vi "Set Module Configuration.vi"(8 "error in (no error)":errorcluster, 10 "Configuration":T2, 11 "Data Cluster":T1) -> (0 "error out":errorcluster, 3 "Data Cluster dup":T1)   [LabVIEW 2014, in "Configurable.lvlib"]
uses:
  Configurable.lvlib
  ModuleConfiguration--Cluster.ctl
  Module Data--cluster.ctl
  <vilib>/LabVIEW Open Source/Configuration Manager/Manager/ConfigManager.lvclass
  <vilib>/LabVIEW Open Source Project/Unicity/UniqueName/UniqueNameClass/UniqueName.lvclass
  <vilib>/LabVIEW Open Source Project/Unicity/UniqueName/UniqueNameClass/UniqueName.lvclass/UniqueName.ctl
  <vilib>/LabVIEW Open Source/Configuration Manager/Manager/ConfigManager.lvclass/ConfigManager.ctl
  <vilib>/LabVIEW Open Source/Configuration Manager/Manager/Write.vi
  <vilib>/LabVIEW Open Source/Configuration Manager/Manager/Read Serializer.vi
  <vilib>/LabVIEW Open Source/Configuration Manager/Manager/Read Encoding.vi
  <vilib>/LabVIEW Open Source/Configuration Manager/Manager/Read Encryption.vi
  <vilib>/LabVIEW Open Source/Configuration Manager/Manager/Decompose KVPs.vi
  <vilib>/Utility/VariantDataType/GetTypeInfo.vi
  <vilib>/LabVIEW Open Source/Configuration Manager/Cache/ConfigManager.Cache.lvclass
  <vilib>/LabVIEW Open Source/Configuration Manager/Serializer/Serializer.lvclass
  <vilib>/LabVIEW Open Source/Configuration Manager/Encoding/Encoding.lvclass
  <vilib>/LabVIEW Open Source/Configuration Manager/Encryption/Encryption.lvclass
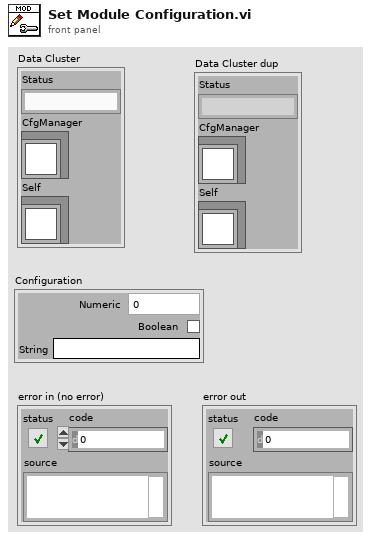
[diagram p1: front panel]
types:
  T1 = typedef "Configurable.lvlib/Module Data--cluster.ctl" = cluster{"Status":string, "CfgManager":refnum<class "ConfigManager.lvclass">, "Self":refnum<class "UniqueName.lvclass">}
  T2 = typedef "Configurable.lvlib/ModuleConfiguration--Cluster.ctl" = cluster{"Numeric":dbl, "Boolean":bool, "String":string}
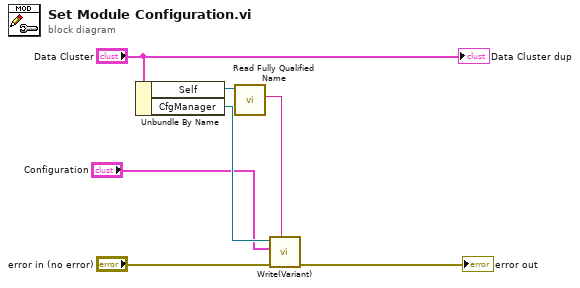
[diagram p0: block diagram]
diagram:
  n1 = Unbundle By Name("Data Cluster") -> ("Self"=w4:refnum<class "UniqueName.lvclass">, "CfgManager"=w5:refnum<class "ConfigManager.lvclass">)
  n2 = call <vilib>:"Read Fully Qualified Name.vi"("UniqueName in"=w4) -> ("Fully Qualified Name"=w6:string)  [unwired: 9 in, 1 out]
  n3 = call <vilib>:"Write(Variant).vi"("Qualified Name"=w6, "error in (no error)"="error in (no error)", "value"="Configuration", "ConfigManager in"=w5) -> ("error out"=→"error out":errorcluster)  [unwired: 5 in, 2 out]
  "Data Cluster dup" <- "Data Cluster"
